vi "例5.12  “按名称解除捆绑”函数.vi"() -> ()   [LabVIEW 2017]
panel:
  out "布尔":bool
  out "字符串":string
  out "簇":cluster{string, i32, bool}={"ABC", 1, FALSE}
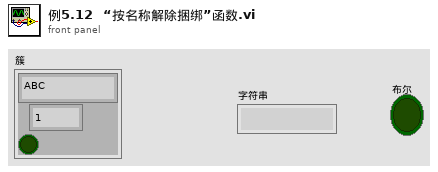
[diagram p1: front panel]
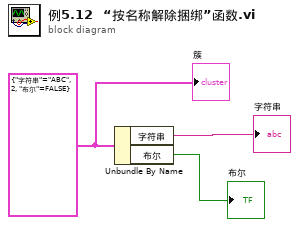
[diagram p0: block diagram]
diagram:
  w3 = cluster{"字符串":string, i32, "布尔":bool} {"字符串"="ABC", 2, "布尔"=FALSE}
  n1 = Unbundle By Name(w3) -> ("字符串"=→"字符串":string, "布尔"=→"布尔":bool)
  "簇" <- w3
